vi "WPI_5865_RobotDriveOpen2MotorWithCANTalonSRX.vi"(5 "Right Motor Inverted":bool, 7 "Left Motor Inverted":bool=TRUE, 8 "error in (no error)":errorcluster, 9 "Control Mode":T1, 10 "Right Motor":u8=20, 11 "Left Motor":u8=10) -> (0 "error out":errorcluster, 3 "RobotDriveDevRef":T2={"DevStatus"={"status"=FALSE, "code"=0, "source"=""}, "Motors[]"=[], "Square Inputs"=FALSE, "Max Output"=1.0})   [LabVIEW 2015]
doc: "Opens a reference to the robot drive for a two-motor robot using CAN TalonSRX motor controllers. The motor controllers are opened in Percent VBus mode.\n\nThis software is licensed. Open the labview\\readme\\WPI Robotics Library Open Source License.txt file for more information."
uses:
  <vilib>/Rock Robotics/WPI/RobotDrive/WPI_RobotDriveDevRef.ctl
  <vilib>/Rock Robotics/WPI/MotorControl/WPI_MotorControlDeviceRef.ctl
  <vilib>/Rock Robotics/WPI/MotorControl/WPI_MotorControlType.ctl
  <vilib>/Rock Robotics/SystemInterfaces/DIO/FPGA_DIOPWMChannel.ctl
  <vilib>/Rock Robotics/WPI/PWM/WPI_PWMDeadband.ctl
  <vilib>/Rock Robotics/WPI/CAN/Jaguar/SubVIs/WPI_CANJaguar_ControlMode.ctl
  <vilib>/Rock Robotics/WPI/CAN/TalonSRX/WPI_CANTalonSRX_APIControlMode.ctl
  <vilib>/Rock Robotics/WPI/SafetyOutput/WPI_SafetyOutputConfigMenu.ctl
  <vilib>/Rock Robotics/WPI/CAN/TalonSRX/WPI_CANTalonSRX_APIFeedbackSelect.ctl
  <vilib>/Rock Robotics/WPI/MotorControl/WPI_MotorControlOpenCANTalonSRX.vi
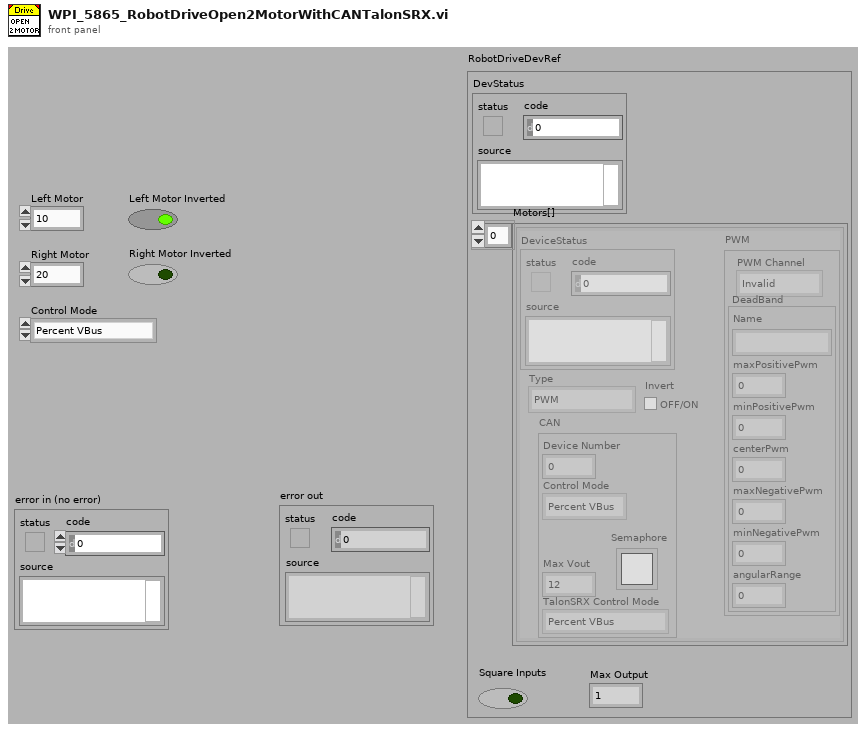
[diagram p1: front panel]
types:
  T1 = typedef "WPI_CANTalonSRX_APIControlMode.ctl" = enum8{"Percent VBus", "Speed", "Position", "Slave", "Unchanged / Invalid", "Voltage Compensation", "Current", "Motion Profile"}
  T2 = typedef "WPI_RobotDriveDevRef.ctl" = cluster{"DevStatus":errorcluster, "Motors[]":T3[], "Square Inputs":bool, "Max Output":dbl}
  T3 = typedef "WPI_MotorControlDeviceRef.ctl" = cluster{"DeviceStatus":errorcluster, "Type":T4, "PWM":cluster{"PWM Channel":T5, "DeadBand":T6}, "CAN":cluster{"Device Number":u8, "Control Mode":T7, "Semaphore":T8, "Max Vout":dbl, "TalonSRX Control Mode":T1}, "Invert":bool}
  T4 = typedef "WPI_MotorControlType.ctl" = enum16{"PWM", "CAN", "CANTalonSRX"}
  T5 = typedef "FPGA_DIOPWMChannel.ctl" = enum8{"PWM 0", "PWM 1", "PWM 2", "PWM 3", "PWM 4", "PWM 5", "PWM 6", "PWM 7", "PWM 8", "PWM 9", "PWM MXP 0", "PWM MXP 1", "PWM MXP 2", "PWM MXP 3", "PWM MXP 4", "PWM MXP 5", "PWM MXP 6", "PWM MXP 7", "PWM MXP 8", "PWM MXP 9", "Invalid"}
  T6 = typedef "WPI_PWMDeadband.ctl" = cluster{"Name":string, "maxPositivePwm":i32, "minPositivePwm":i32, "centerPwm":i32, "maxNegativePwm":i32, "minNegativePwm":i32, "angularRange":u16}
  T7 = typedef "WPI_CANJaguar_ControlMode.ctl" = enum8{"Percent VBus", "Current", "Speed", "Position", "Voltage"}
  T8 = typedef "Semaphore RefNum" = refnum<k1>
  T9 = typedef "WPI_SafetyOutputConfigMenu.ctl" = enum16{"Enable", "Disable"}
  T10 = typedef "WPI_CANTalonSRX_APIFeedbackSelect.ctl" = enum16{"Digital Quadrature Encoder", "Analog Potentiometer", "Analog Encoder", "Count on Quad-A (Rising-Edge)", "Count on Quad-A (Falling-Edge)", "CTR Magnetic Enc (Absolute)", "CTR Magnetic Enc (Relative)", "Pulse Width"}
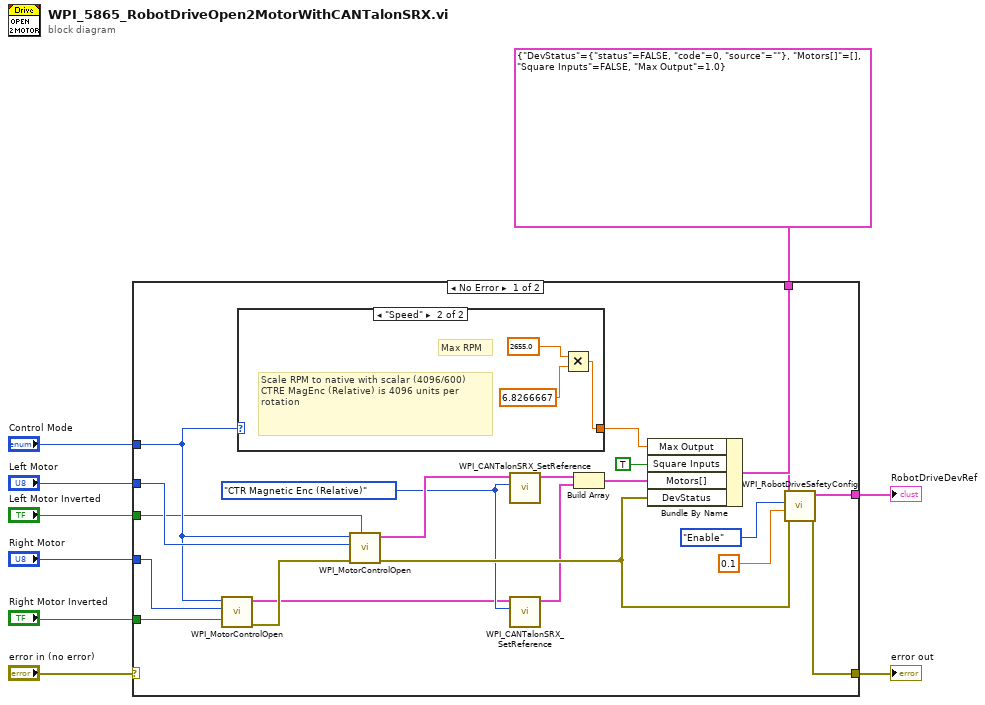
[diagram p0: block diagram]
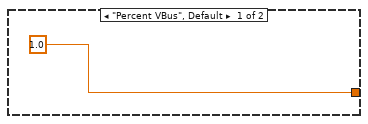
[diagram p2: hidden frame]
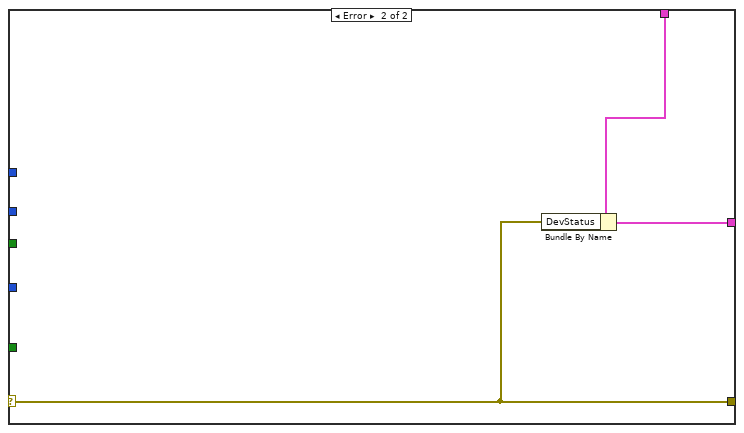
[diagram p3: hidden frame]
diagram:
  n1 = case shown="No Error" "error in (no error)" {
    selector: "error in (no error)" -> [_ w35]
    tunnel: "Left Motor" -> [w22 _]
    tunnel: "Right Motor" -> [w21 _]
    tunnel: [w20 w37] -> w7
    tunnel: "Left Motor Inverted" -> [w13 _]
    tunnel: "Right Motor Inverted" -> [w12 _]
    tunnel: T2 {"DevStatus"={"status"=FALSE, "code"=0, "source"=""}, "Motors[]"=[], "Square Inputs"=FALSE, "Max Output"=1.0} ("RobotDriveDevRef") -> [w29 w36]
    tunnel: [w23 w35] -> w2
    tunnel: "Control Mode" -> [w17 _]
    frame No Error {
      w11 = WPI_CANTalonSRX_APIFeedbackSelect."CTR Magnetic Enc (Relative)" ("Feedback Reference")
      n2 = call-poly <vilib>:"WPI_MotorControlOpen.vi"("Invert"=w12, "Device Number"=w21, "Control Mode"=w17) -> ("error out"=w27:errorcluster, "MotorControlDeviceRef"=w10:T3)  [unwired: 2 in, 5 out]
      n3 = case shown="\"Speed\"" w17 {
        tunnel: [1.0 ("Max Output") w33] -> w19
        frame "Percent VBus", Default {
        }
        frame "Speed" {
          # "Scale RPM to native with scalar (4096/600)\nCTRE MagEnc (Relative) is 4096 units per rotation"
          # "Max RPM"
          n4 = Multiply(x=2655.0 ("Max Output"), y=6.8266667) -> (x*y=w33:dbl)
        }
      }
      n5 = call-poly <vilib>:"WPI_MotorControlOpen.vi"("Invert"=w13, "error in (no error)"=w27, "Device Number"=w22, "Control Mode"=w17) -> ("error out"=w24:errorcluster, "MotorControlDeviceRef"=w15:T3)  [unwired: 1 in, 5 out]
      n6 = call <vilib>:"WPI_CANTalonSRX_SetReference.vi"("Feedback Reference"=w11, "CAN Talon SRX Ref"=w15) -> ("CAN Talon SRX Ref"=w14:T3)  [unwired: 8 in, 1 out]
      n7 = call <vilib>:"WPI_CANTalonSRX_SetReference.vi"("Feedback Reference"=w11, "CAN Talon SRX Ref"=w10) -> ("CAN Talon SRX Ref"=w16:T3)  [unwired: 8 in, 1 out]
      n8 = Build Array(w14, w16) -> (w30:T3[])
      n9 = Bundle By Name(cluster=w29, "Max Output"=w19, "Square Inputs"=TRUE ("DestroyPWM?"), "Motors[]"=w30, "DevStatus"=w24) -> (w26:T2)
      n10 = call <vilib>:"WPI_RobotDriveSafetyConfig.vi"("error in (no error)"=w24, "timeout (s)"=0.1, "mode"=WPI_SafetyOutputConfigMenu."Enable", "RobotDriveDevRef"=w26) -> ("error out"=w23:errorcluster, "RobotDriveDevRef"=w20:T2)  [unwired: 6 out]
    }
    frame Error {
      n11 = Bundle By Name(cluster=w36, "DevStatus"=w35) -> (w37:T2)
    }
  }
  "RobotDriveDevRef" <- w7
  "error out" <- w2
